vi "Main.vi"() -> ()   [LabVIEW 2019]
uses:
  <resource>/objmgr/daqmx.rc
panel:
  in  "Exit Button":bool
  in  "Analyze Button":bool
  in  "Calibrate Button":bool
  in  "Collect Button":bool
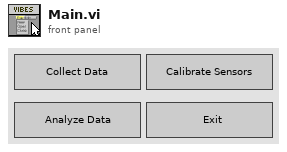
[diagram p1: front panel]
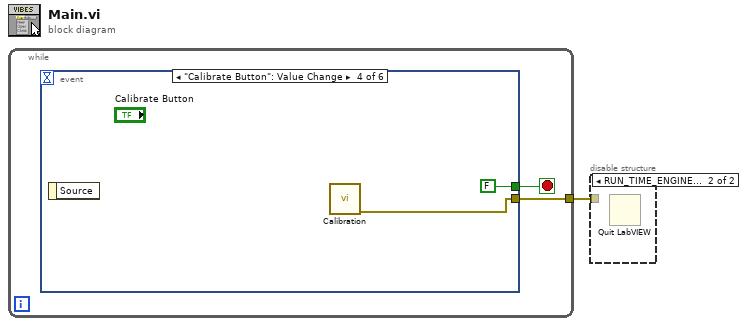
[diagram p0: block diagram]
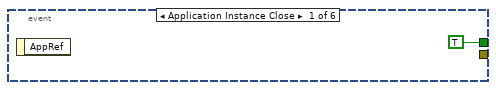
[diagram p3: hidden frame]
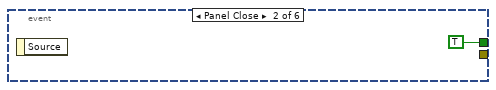
[diagram p4: hidden frame]
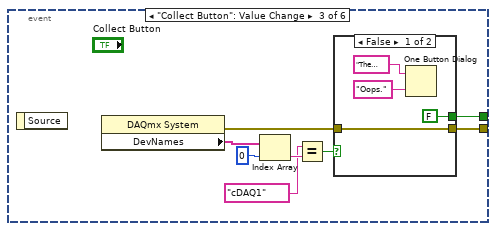
[diagram p5: hidden frame]
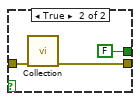
[diagram p6: hidden frame]
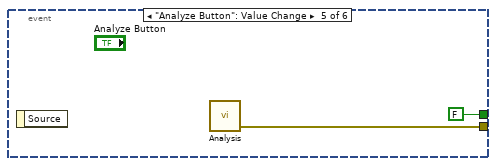
[diagram p7: hidden frame]
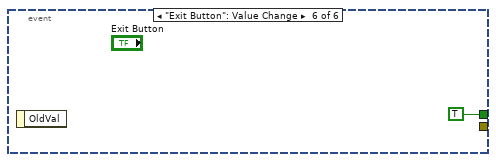
[diagram p8: hidden frame]
diagram:
  n1 = while {
    tunnel: [w2] -> w1
    stop <- w3 stop-if-true
    n2 = event shown="[3] \"Calibrate Button\": Value Change" {
      selector: _ -> [_ _ _ _ _ _]
      dyn-events: _ -> [_ _ _ _ _ _]
      timeout: _ -> [_ _ _ _ _ _]
      tunnel: [TRUE TRUE w13 FALSE FALSE TRUE] -> w3
      tunnel: [_ _ w12 w21 w23 _] -> w2
      event Application Instance Close {
        n3 = event-data() -> ()  [unwired: 1 in, 1 out]
      }
      event Panel Close {
        n4 = event-data() -> ()  [unwired: 1 in, 1 out]
      }
      event "Collect Button": Value Change {
        n5 = event-data() -> ()  [unwired: 1 in, 1 out]
        n6 = property class="DAQmx System"() -> (error out=w6:errorcluster, "DevNames"=w11:tag[])  [unwired: 2 in, 1 out]
        n7 = Index Array(array=w11, index=0) -> (element=w9:tag)
        n8 = Equal?(x=tag "cDAQ1", y=w9) -> (x = y?=w7:bool)
        n9 = case shown="False" w7 {
          tunnel: [FALSE FALSE] -> w13
          tunnel: [w14 w19] -> w12
          tunnel: w6 -> [w14 w18]
          frame False {
            n10 = One Button Dialog(message="The DAQ board is not plugged in", button name ("OK")="Oops.") -> ()  [unwired: 1 out]
          }
          frame True {
            n11 = call "Collection.vi"("error in (no error)"=w18) -> ("error out"=w19:errorcluster)  [unwired: 10 in]
          }
        }
      }
      event "Calibrate Button": Value Change {
        n12 = event-data() -> ()  [unwired: 1 in, 1 out]
        n13 = call "Calibration.vi"() -> ("Error Out"=w21:errorcluster)  [unwired: 11 in]
      }
      event "Analyze Button": Value Change {
        n14 = event-data() -> ()  [unwired: 1 in, 1 out]
        n15 = call "Analysis.vi"() -> ("error out"=w23:errorcluster)  [unwired: 11 in]
      }
      event "Exit Button": Value Change {
        n16 = event-data() -> ()  [unwired: 1 in, 1 out]
      }
    }
  }
  n17 = disable-structure shown="RUN_TIME_ENGINE==True" {
    disable-tunnel: w1 -> [_ _]
    frame condition #0 (active) {
    }
    frame condition #1 {
      n18 = Quit LabVIEW() -> ()  [unwired: 1 in]
    }
  }
